vi "Eliminar ceros dentro de while.vi"() -> ()   [LabVIEW 2016]
panel:
  out "reversed array 2":dbl[](array[numeric])
  out "reversed array":dbl[](array[numeric])
  out "appended array":dbl[](array[numeric])
  in  "stop":bool
  out "element":dbl
  in  "array":dbl[](array[numeric])=[3.0, 4.0, 0.0, 0.0, 2.0, 35.0, 0.0, 32.0, 0.0, 0.0, 12.0, 8.0, 6.0, 0.0, 2.0]
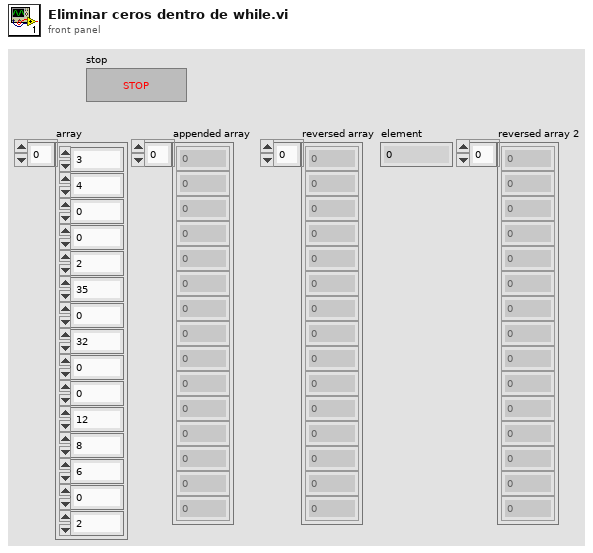
[diagram p1: front panel]
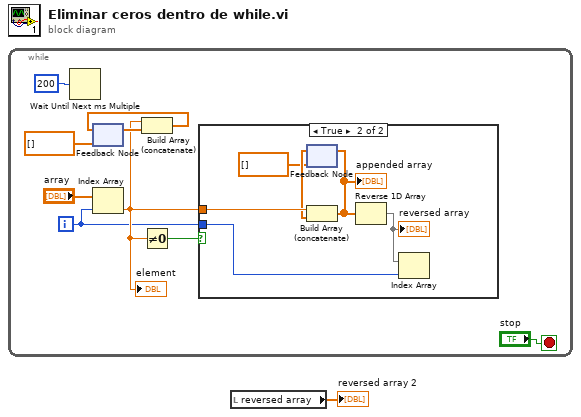
[diagram p0: block diagram]
diagram:
  n1 = while {
    i -> [w2]
    stop <- "stop" stop-if-true
    n2 = Wait Until Next ms Multiple(millisecond multiple=u32 200) -> ()  [unwired: 1 out]
    n3 = feedback #1(dbl[] []) -> (w5:dbl[])
    n4 = Index Array(array="array", index=w2) -> (element=w3:dbl)
    "element" <- w3
    n5 = Build Array (concatenate)(w3, w5) -> (w7:dbl[])
    n6 = feedback-in #1(w7) -> ()
    n7 = Not Equal To 0?(x=w3) -> (x != 0?=w4:bool)
    n8 = case shown="True" w4 {
      tunnel: w3 -> [_ w16]
      tunnel: w2 -> [_ w11]
      frame False {
      }
      frame True {
        n9 = feedback #2(dbl[] []) -> (w15:dbl[])
        n10 = Build Array (concatenate)(w16, w15) -> (w13:dbl[])
        "appended array" <- w13
        n11 = feedback-in #2(w13) -> ()
        n12 = Reverse 1D Array(array=w13) -> (reversed array=w12:dbl[])
        "reversed array" <- w12
        n13 = Index Array(array=w12, index=w11) -> ()  [unwired: 1 out]
      }
    }
  }
  n14 = local read "reversed array"() -> (→"reversed array 2":dbl[])
